vi "Test_AddGetTopic_RetrievalOK.vi"(8 "error in (no error)":errorcluster, 11 "TestCase in":refnum<class "TestTopicLookupTable.lvclass">) -> (0 "error out":errorcluster, 3 "TestCase out":refnum<class "TestTopicLookupTable.lvclass">)   [LabVIEW 2017, in "TestTopicLookupTable.lvclass"]
uses:
  TestTopicLookupTable.lvclass
  <vilib>/ActorFramework/Message Queue/Message Queue.lvclass/Message Queue.ctl
  Topic/Topic.lvclass/Topic.ctl
  TopicLookupTable/TopicLookupTable.lvclass/TopicLookupTable.ctl
  Topic/Read Topic Info.vi
  <vilib>/ActorFramework/Actor/Read Self Enqueuer.vi
  <vilib>/ActorFramework/Message Enqueuer/Init from Existing Queue.vi
  gpm_packages/@cs/variant/Source/Format Type String.vi
  <vilib>/ActorFramework/Message Enqueuer/Message Enqueuer.lvclass
  <vilib>/addons/_JKI Toolkits/VI Tester/TestCase.llb/TestCase.lvclass
  TopicLookupTable/TopicLookupTable.lvclass
  Topic/Topic.lvclass
  <vilib>/ActorFramework/Message Queue/Message Queue.lvclass
  C:/Program Files (x86)/National Instruments/LabVIEW 2017/vi.lib/addons/_JKI Toolkits/VI Tester/TestCase.llb/TestCase.lvclass
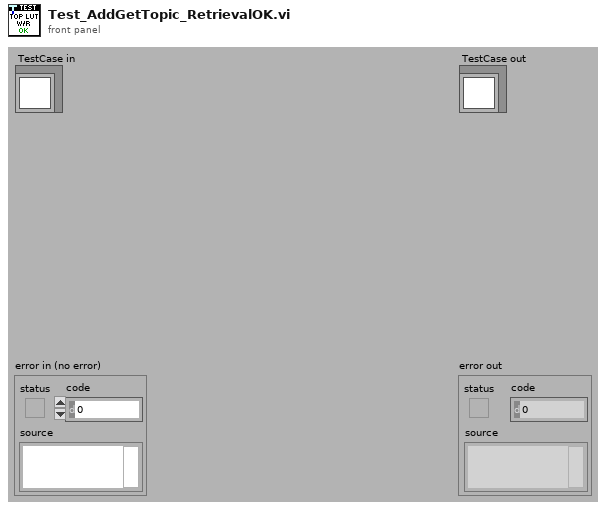
[diagram p1: front panel]
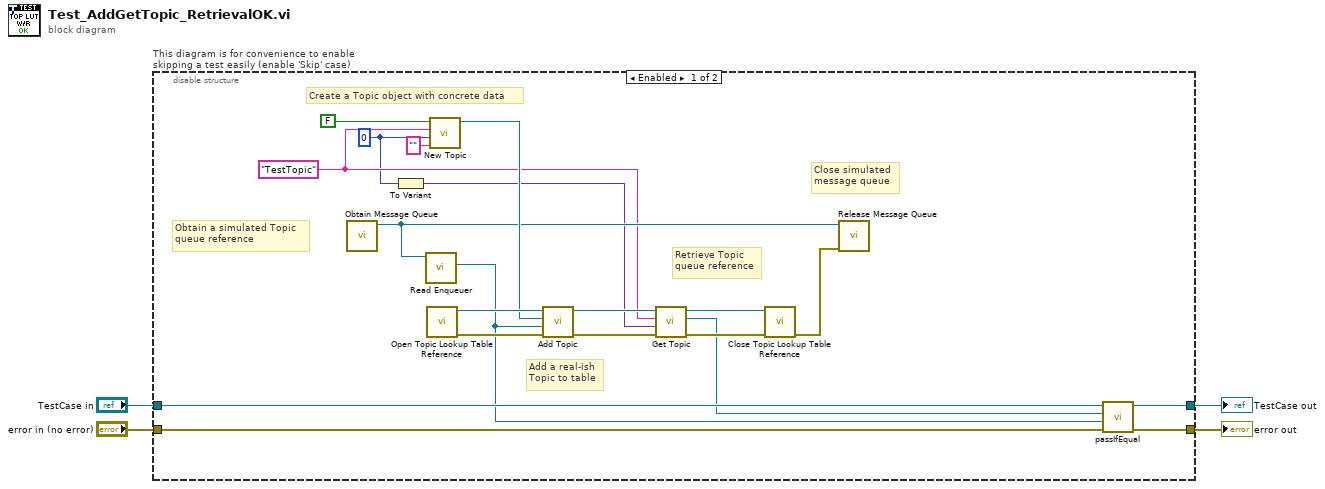
[diagram p0: block diagram]
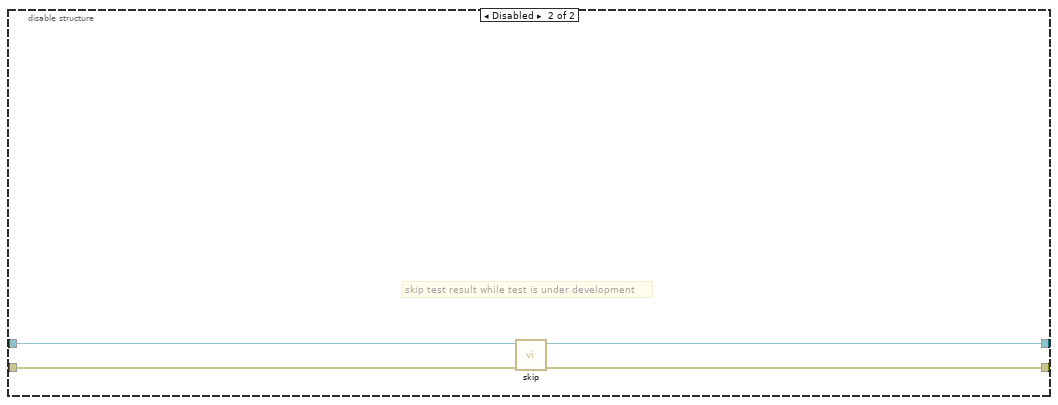
[diagram p2: hidden frame]
diagram:
  n1 = disable-structure "This diagram is for convenience to enable skipping a test easily (enable 'Skip' case)" shown="Enabled" {
    disable-tunnel: "TestCase in" -> [w24 w28]
    disable-tunnel: [w23 w26] -> w1
    disable-tunnel: [w22 w27] -> w3
    disable-tunnel: "error in (no error)" -> [w21 w25]
    frame Enabled {
      w9 = 0
      w10 = "TestTopic" ("Name")
      # "Create a Topic object with concrete data"
      # "Add a real-ish\nTopic to table"
      # "Close simulated\nmessage queue"
      # "Retrieve Topic\nqueue reference"
      # "Obtain a simulated Topic\nqueue reference"
      n2 = call <vilib>:"Obtain Message Queue.vi"() -> ("Message Queue"=w11:refnum<class "Message Queue.lvclass">)  [unwired: 10 in, 1 out]
      n3 = To Variant(anything=w9) -> (Variant=w8:variant)
      n4 = call <vilib>:"Read Enqueuer.vi"("Message Queue"=w11) -> ("Message Enqueuer"=w13:refnum<class "Message Enqueuer.lvclass">)  [unwired: 10 in]
      n5 = call "Open Topic Lookup Table Reference.vi"() -> ("error out"=w19:errorcluster, "TopicLookupTable Reference"=w20:refnum<data-value>)  [unwired: 10 in]
      n6 = call "New Topic.vi"("Lock Owner ID (\"\" = NOT Locked)"="" ("Lock Owner ID (\"\" = NOT Locked)"), "New Topic Data"=w9, "Name"=w10, "Use Type Input As Initial Value?"=FALSE) -> ("Topic out"=w14:refnum<class "Topic.lvclass">)  [unwired: 6 in, 1 out]
      n7 = call "Add Topic.vi"("error in (no error)"=w19, "Topic Enqueuer"=w13, "Topic Object"=w14, "TopicLookupTable"=w20) -> ("error out"=w17:errorcluster, "TopicLookupTable"=w18:refnum<data-value>)  [unwired: 5 in, 1 out]
      n8 = call "Get Topic.vi"("error in (no error)"=w17, "Topic Type"=w8, "Topic Name"=w10, "TopicLookupTable"=w18) -> ("error out"=w15:errorcluster, "Topic Enqueuer"=w7:refnum<class "Message Enqueuer.lvclass">, "TopicLookupTable"=w16:refnum<data-value>)  [unwired: 5 in]
      n9 = call "Close Topic Lookup Table Reference.vi"("error in (no error)"=w15, "TopicLookupTable"=w16) -> ("error out"=w12:errorcluster)  [unwired: 9 in]
      n10 = call <vilib>:"Release Message Queue.vi"("error in (no error)"=w12, "Message Queue"=w11) -> ()  [unwired: 8 in, 2 out]
      n11 = call-dynamic "passIfEqual.vi"("error in (no error)"=w21, "y"=w13, "x"=w7, "TestCase in"=w24) -> ("error out"=w22:errorcluster, "TestCase out"=w23:refnum<class "TestTopicLookupTable.lvclass">)  [unwired: 6 in]
    }
    frame Disabled {
      # "skip test result while test is under development"
      n12 = call <vilib>:"skip.vi"("error in (no error)"=w25, "TestCase in"=w28) -> ("error out"=w27:errorcluster, "TestCase out"=w26:refnum<class "TestTopicLookupTable.lvclass">)  [unwired: 8 in]
    }
  }
  "error out" <- w3
  "TestCase out" <- w1
